vi "czytajI2C.vi"(7 "I2C Channel":u8, 8 "Error In":errorcluster, 9 "Czy uśrednić?":bool, 10 "I2C Slave Address (0x1D)":u8, 11 "LINX Resource in":T1) -> (0 "Error Out":errorcluster, 1 "Czy kolejka pełna?":bool, 2 "Acceleration Data (g)":T7, 3 "LINX Resource out":T1, 4 "kąt nachylenia":dbl)   [LabVIEW 2014]
uses:
  <vilib>/MakerHub/LINX/LMH-LINX.lvlib
  czytajI2CVIs/usrednijVIs/AkcjaUsredniania.ctl
  <vilib>/MakerHub/LINX/Private/Type Defs/Platform.ctl
  <vilib>/MakerHub/LINX/Private/Type Defs/Interface.ctl
  <vilib>/MakerHub/LINX/Private/Device/Type Defs/TCP Config.ctl
  <vilib>/MakerHub/LINX/Private/Device/Device.lvlib
  <vilib>/MakerHub/LINX/Private/Device/Type Defs/Channels.ctl
  <vilib>/MakerHub/LINX/Private/Device/Type Defs/LINX Device Config.ctl
  <vilib>/MakerHub/LINX/Private/Type Defs/LINX Ref.ctl
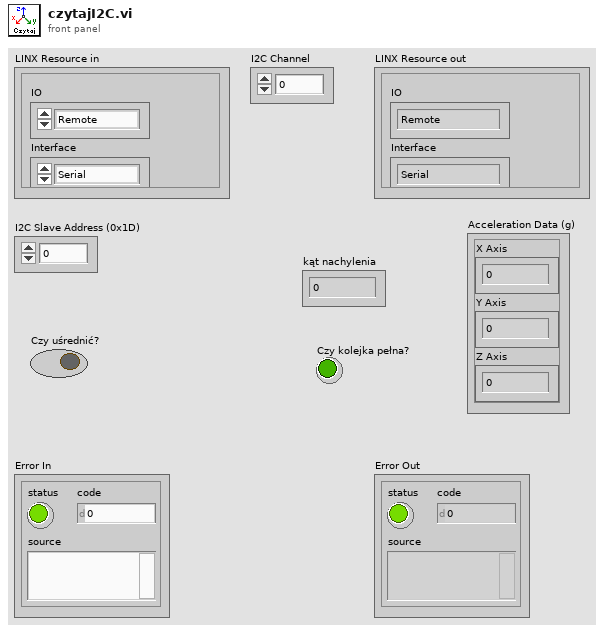
[diagram p1: front panel]
types:
  T1 = typedef "LMH-LINX.lvlib/LINX Ref.ctl" = cluster{"IO":T2, "Interface":T3, "LINX Device Config":T4}
  T2 = typedef "LMH-LINX.lvlib/Platform.ctl" = enum16{"Remote", "Local"}
  T3 = typedef "LMH-LINX.lvlib/Interface.ctl" = enum16{"Serial", "TCP"}
  T4 = typedef "LMH-LINX.lvlib/Device.lvlib/LINX Device Config.ctl" = cluster{"Interface":T3, "COM Port":refnum<visa-resource-name>, "TCP Configuration":T5, "Device Family":u8, "Device ID":u8, "Device Name":string, "TCP Ref":refnum<k5>, "Channels":T6}
  T5 = typedef "LMH-LINX.lvlib/Device.lvlib/TCP Config.ctl" = cluster{"IP Address":string, "Port":u16}
  T6 = typedef "LMH-LINX.lvlib/Channels.ctl" = cluster{"DI":u8[], "DO":u8[], "AI":u8[], "AO":u8[], "PWM":u8[], "QE":u8[], "UART":u8[], "I2C 2":u8[], "SPI":u8[], "CAN":u8[], "Servo":u8[], "AI Ref (V)":dbl, "AI Resolution (Bits)":u8, "AO Ref (V)":dbl, "AO Resolution (Bits)":u8}
  T7 = cluster{"X Axis":dbl, "Y Axis":dbl, "Z Axis":dbl}
  T8 = typedef "AkcjaUsredniania.ctl" = enum16{"Init", "DodajWartość", "WypełnijKolejkę", "Czyść"}
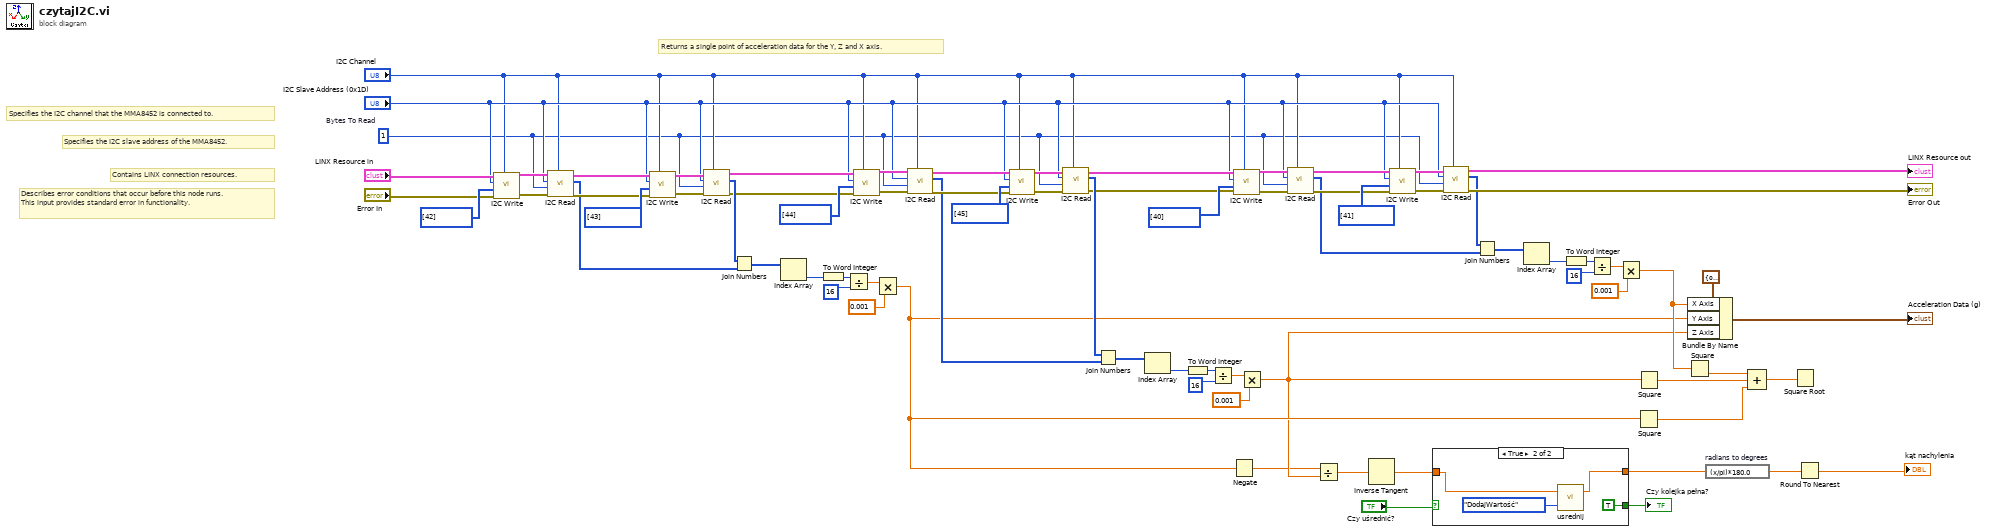
[diagram p0: block diagram]
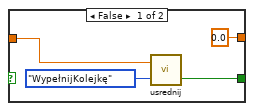
[diagram p2: hidden frame]
diagram:
  w24 = u8 1  # Bytes To Read
  # "Returns a single point of acceleration data for the Y, Z and X axis."
  # "Specifies the I2C slave address of the MMA8452."
  # "Specifies the I2C channel that the MMA8452 is connected to."
  # "Contains LINX connection resources."
  # "Describes error conditions that occur before this node runs. This input provides standard error in functionality."
  n1 = call <vilib>:"I2C Write.vi"("I2C Channel"="I2C Channel", "Error In"="Error In", "Data"=u8[] [42], "I2C Slave Address (0)"="I2C Slave Address (0x1D)", "LINX Resource"="LINX Resource in") -> ("Error Out"=w74:errorcluster, "LINX Resource"=w75:T1)  [unwired: 5 in]
  n2 = call <vilib>:"I2C Read.vi"("I2C Channel"="I2C Channel", "Error In"=w74, "Bytes To Read"=w24, "I2C Slave Address (0)"="I2C Slave Address (0x1D)", "LINX Resource"=w75) -> ("Error Out"=w61:errorcluster, "Data"=w57:u8[], "LINX Resource"=w62:T1)  [unwired: 4 in]
  n3 = call <vilib>:"I2C Write.vi"("I2C Channel"="I2C Channel", "Error In"=w61, "Data"=u8[] [43], "I2C Slave Address (0)"="I2C Slave Address (0x1D)", "LINX Resource"=w62) -> ("Error Out"=w63:errorcluster, "LINX Resource"=w60:T1)  [unwired: 5 in]
  n4 = call <vilib>:"I2C Read.vi"("I2C Channel"="I2C Channel", "Error In"=w63, "Bytes To Read"=w24, "I2C Slave Address (0)"="I2C Slave Address (0x1D)", "LINX Resource"=w60) -> ("Error Out"=w47:errorcluster, "Data"=w58:u8[], "LINX Resource"=w48:T1)  [unwired: 4 in]
  n5 = Join Numbers(hi=w58, lo=w57) -> ((hi.lo)=w59:u16[])
  n6 = Index Array(array=w59) -> (element=w71:u16)  [unwired: 1 in]
  n7 = To Word Integer(number=w71) -> (16bit integer=w70:i16)
  n8 = Divide(x=w70, y=i16 16) -> (x/y=w68:dbl)
  n9 = call <vilib>:"I2C Write.vi"("I2C Channel"="I2C Channel", "Error In"=w47, "Data"=u8[] [44], "I2C Slave Address (0)"="I2C Slave Address (0x1D)", "LINX Resource"=w48) -> ("Error Out"=w54:errorcluster, "LINX Resource"=w55:T1)  [unwired: 5 in]
  n10 = Multiply(x=w68, y=0.001) -> (x*y=w8:dbl)
  n11 = call <vilib>:"I2C Read.vi"("I2C Channel"="I2C Channel", "Error In"=w54, "Bytes To Read"=w24, "I2C Slave Address (0)"="I2C Slave Address (0x1D)", "LINX Resource"=w55) -> ("Error Out"=w50:errorcluster, "Data"=w40:u8[], "LINX Resource"=w51:T1)  [unwired: 4 in]
  n12 = call <vilib>:"I2C Write.vi"("I2C Channel"="I2C Channel", "Error In"=w50, "Data"=u8[] [45], "I2C Slave Address (0)"="I2C Slave Address (0x1D)", "LINX Resource"=w51) -> ("Error Out"=w52:errorcluster, "LINX Resource"=w49:T1)  [unwired: 5 in]
  n13 = call <vilib>:"I2C Read.vi"("I2C Channel"="I2C Channel", "Error In"=w52, "Bytes To Read"=w24, "I2C Slave Address (0)"="I2C Slave Address (0x1D)", "LINX Resource"=w49) -> ("Error Out"=w29:errorcluster, "Data"=w39:u8[], "LINX Resource"=w30:T1)  [unwired: 4 in]
  n14 = Join Numbers(hi=w39, lo=w40) -> ((hi.lo)=w41:u16[])
  n15 = Index Array(array=w41) -> (element=w46:u16)  [unwired: 1 in]
  n16 = To Word Integer(number=w46) -> (16bit integer=w45:i16)
  n17 = Divide(x=w45, y=i16 16) -> (x/y=w43:dbl)
  n18 = Negate(x=w8) -> (-x=w6:dbl)
  n19 = call <vilib>:"I2C Write.vi"("I2C Channel"="I2C Channel", "Error In"=w29, "Data"=u8[] [40], "I2C Slave Address (0)"="I2C Slave Address (0x1D)", "LINX Resource"=w30) -> ("Error Out"=w36:errorcluster, "LINX Resource"=w37:T1)  [unwired: 5 in]
  n20 = Multiply(x=w43, y=0.001) -> (x*y=w7:dbl)
  n21 = call <vilib>:"I2C Read.vi"("I2C Channel"="I2C Channel", "Error In"=w36, "Bytes To Read"=w24, "I2C Slave Address (0)"="I2C Slave Address (0x1D)", "LINX Resource"=w37) -> ("Error Out"=w32:errorcluster, "Data"=w16:u8[], "LINX Resource"=w33:T1)  [unwired: 4 in]
  n22 = Divide(x=w6, y=w7) -> (x/y=w5:dbl)
  n23 = Inverse Tangent(1:w5) -> (0:w4:dbl)
  n24 = call <vilib>:"I2C Write.vi"("I2C Channel"="I2C Channel", "Error In"=w32, "Data"=u8[] [41], "I2C Slave Address (0)"="I2C Slave Address (0x1D)", "LINX Resource"=w33) -> ("Error Out"=w34:errorcluster, "LINX Resource"=w31:T1)  [unwired: 5 in]
  n25 = case shown="True" "Czy uśrednić?" {
    tunnel: w4 -> [w80 w83]
    tunnel: [0.0 ("Przysp. uśrednione") w82] -> w3
    tunnel: [w77 TRUE ("Czy kolejka pełna?")] -> w1
    frame False {
      n26 = call "usrednij.vi"("AkcjaUsredniania"=AkcjaUsredniania."WypełnijKolejkę", "Wartość"=w80) -> ("Czy kolejka pełna?"=w77:bool)  [unwired: 1 out]
    }
    frame True {
      n27 = call "usrednij.vi"("AkcjaUsredniania"=AkcjaUsredniania."DodajWartość", "Wartość"=w83) -> ("Przysp. uśrednione"=w82:dbl)  [unwired: 1 out]
    }
  }
  "Czy kolejka pełna?" <- w1
  n28 = call <vilib>:"I2C Read.vi"("I2C Channel"="I2C Channel", "Error In"=w34, "Bytes To Read"=w24, "I2C Slave Address (0)"="I2C Slave Address (0x1D)", "LINX Resource"=w31) -> ("Error Out"=→"Error Out":errorcluster, "Data"=w17:u8[], "LINX Resource"=→"LINX Resource out":T1)  [unwired: 4 in]
  n29 = Join Numbers(hi=w17, lo=w16) -> ((hi.lo)=w18:u16[])
  n30 = Index Array(array=w18) -> (element=w23:u16)  [unwired: 1 in]
  n31 = To Word Integer(number=w23) -> (16bit integer=w22:i16)
  n32 = Divide(x=w22, y=i16 16) -> (x/y=w20:dbl)
  n33 = Multiply(x=w20, y=0.001) -> (x*y=w15:dbl)
  n34 = Square(x=w8) -> (x^2=w12:dbl)
  n35 = Square(x=w7) -> (x^2=w13:dbl)
  n36 = Square(x=w15) -> (x^2=w14:dbl)
  n37 = Bundle By Name(cluster=T7 {"X Axis"=0.0, "Y Axis"=0.0, "Z Axis"=0.0} ("Acceleration Data (g)"), "X Axis"=w15, "Y Axis"=w8, "Z Axis"=w7) -> (→"Acceleration Data (g)":T7)
  n38 = expression code="(x/pi)*180.0" "radians to degrees"(w3) -> (w10:dbl)
  n39 = Compound Arithmetic op=ADD(w14, w13, w12) -> (w11:dbl)
  n40 = Square Root(x=w11) -> ()  [unwired: 1 out]
  n41 = Round To Nearest(number=w10) -> (nearest integer value=→"kąt nachylenia":dbl)
